vi "Loops_001.vi"() -> ()   [LabVIEW 2019]
panel:
  out "instantaneous Number of iterations 2":i32
  out "Number of iterations":i32
  in  "stop":bool
  in  "Slide":dbl(slide) scale=0.0..10.0
  out "Waveform Chart":dbl(graph)
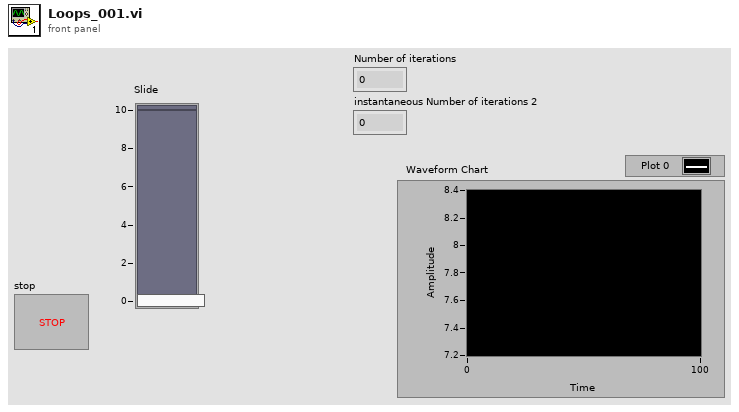
[diagram p1: front panel]
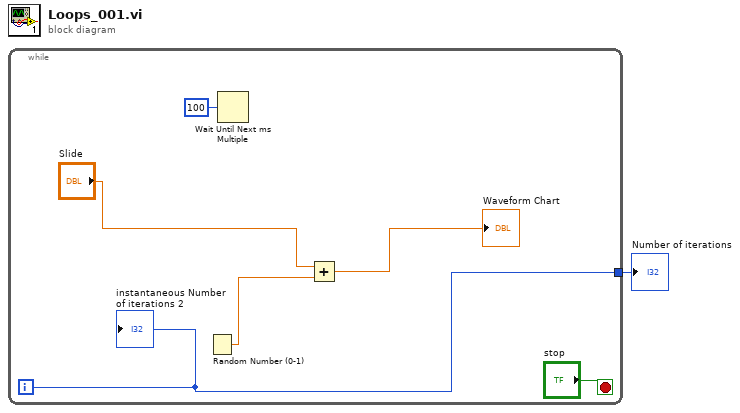
[diagram p0: block diagram]
diagram:
  n1 = while {
    tunnel: [w2] -> w1
    i -> [w2]
    stop <- "stop" stop-if-true
    n2 = Random Number (0-1)() -> (number: 0 to 1=w3:dbl)
    n3 = Wait Until Next ms Multiple(millisecond multiple=u32 100) -> ()  [unwired: 1 out]
    n4 = Add(x="Slide", y=w3) -> (x+y=→"Waveform Chart":dbl)
    "instantaneous Number of iterations 2" <- w2
  }
  "Number of iterations" <- w1
